vi "ReadTerminals.vi"() -> ()   [LabVIEW 2018]
uses:
  <instrlib>/BK Precision 85XX Series/BK Precision 85XX Series.lvlib
panel:
  out "Terminal Input Power (W)":dbl(knob) scale=0.0..5000.0 scale format="%#_3f"
  out "Terminal Input Current (A)":dbl(knob) scale=0.0..240.0 scale format="%#_3g"
  out "Terminal Input Voltage (V)":dbl(knob) scale=0.0..5.0 scale format="%#_3g"
  in  "Communication Address (0)":u8 max=254 format="%x"
  in  "Serial Configuration":T1={"Baud Rate"=9600, "Parity"=0, "Data Bits"=8, "Stop Bits"=10} {"Stop Bits" items=["1.0"=10]; "Data Bits" items=["8"=8]; "Parity" items=["None", "Odd", "Even"]; "Baud Rate" items=["4800"=4800, "9600"=9600, "19200"=19200, "38400"=38400]}
  in  "VISA resource name":refnum<visa-resource-name>
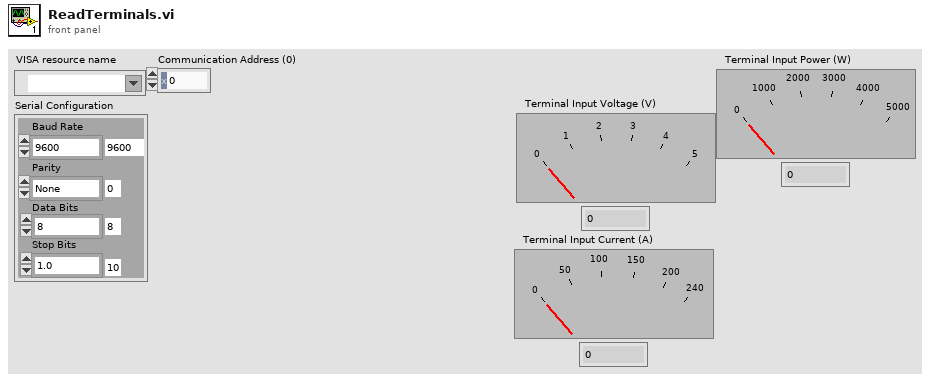
[diagram p1: front panel]
types:
  T1 = cluster{"Baud Rate":u32, "Parity":u16, "Data Bits":u16, "Stop Bits":u16}
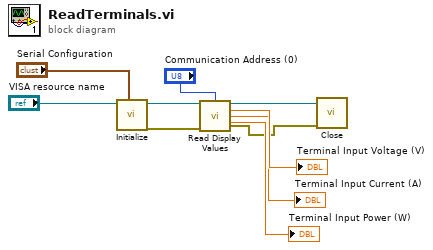
[diagram p0: block diagram]
diagram:
  n1 = call <instrlib>:"Initialize.vi"("Serial Configuration"="Serial Configuration", "VISA resource name"="VISA resource name") -> ("error out"=w7:errorcluster, "VISA resource name out"=w8:refnum<visa-resource-name>)  [unwired: 8 in]
  n2 = call <instrlib>:"Read Display Values.vi"("VISA resource name"=w8, "Communication Address (0)"="Communication Address (0)", "error in (no error)"=w7) -> ("VISA resource name out"=w2:refnum<visa-resource-name>, "Terminal Input Voltage (V)"=→"Terminal Input Voltage (V)":dbl, "Terminal Input Current (A)"=→"Terminal Input Current (A)":dbl, "Terminal Input Power (W)"=→"Terminal Input Power (W)":dbl, "error out"=w1:errorcluster)  [unwired: 8 in]
  n3 = call <instrlib>:"Close.vi"("error in (no error)"=w1, "VISA resource name"=w2) -> ()  [unwired: 9 in, 1 out]
